vi "Sensor Calibration.vi"(5 "Error In":errorcluster) -> (15 "SubGP Slope":dbl, 16 "SubGP Intercept":dbl, 17 "Flow Slope":dbl, 18 "Flow Intercept":dbl, 19 "Error Out":errorcluster)   [LabVIEW 2020, in "MainVIs.lvlib"]
uses:
  MainVIs.lvlib
  <vilib>/Analysis/baseanly.llb/Mean (DBL).vi
  <vilib>/Analysis/NI_AALBase.lvlib
  SubVIs.lvlib
panel:
  out "SupraGP Slope":dbl
  out "SupraGP Intercept":dbl
  out "SupraGP Voltage":dbl
  out "Flow Voltage":dbl
  in  "Add Button HS":bool
  in  "Stop Button HS":bool
  out "SubGP Voltage":dbl
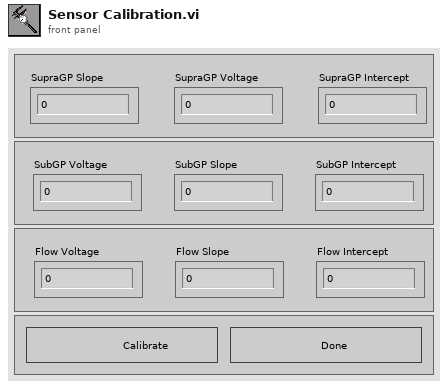
[diagram p1: front panel]
types:
  T1 = enum8{"Enabled", "Disabled", "Disabled and Grayed Out"}
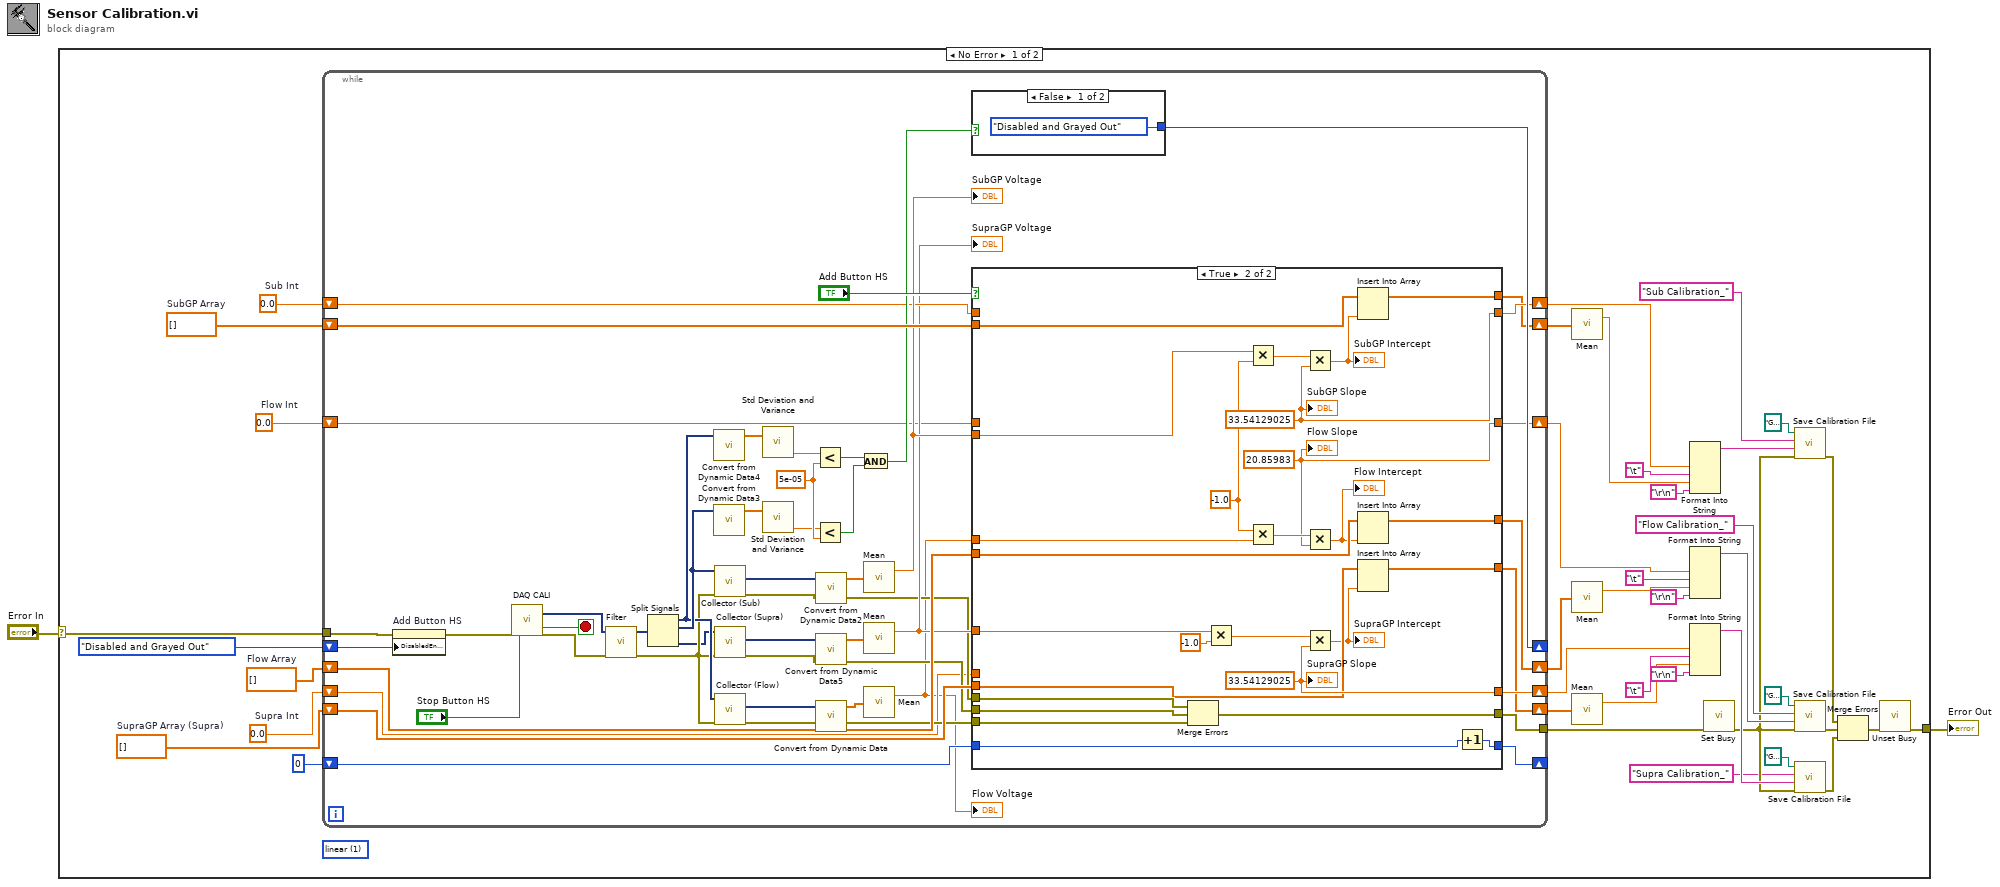
[diagram p0: block diagram]
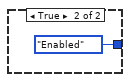
[diagram p2: hidden frame]
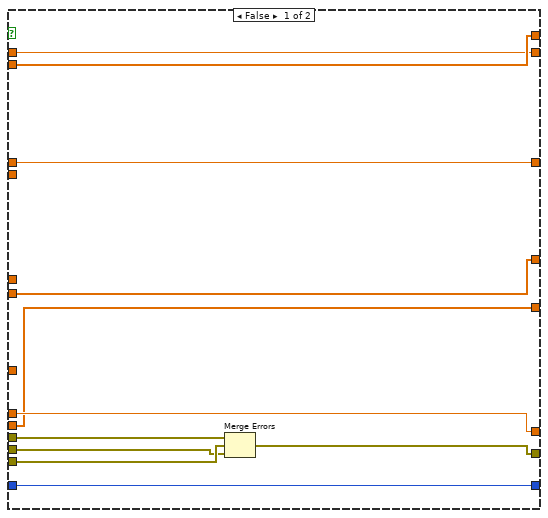
[diagram p3: hidden frame]
diagram:
  n1 = case shown="No Error" "Error In" {
    selector: "Error In" -> [w13 w131]
    tunnel: [w35 w131] -> w2
    frame No Error {
      w4 = 0.0  # Supra Int
      w11 = 0.0  # Flow Int
      w14 = 0.0  # Sub Int
      w17 = dbl[] []  # SupraGP Array (Supra)
      w40 = dbl[] []  # SubGP Array
      (unwired) 1 items=["nearest", "linear", "spline", "cubic Hermite", "Lagrange"] ("method")
      w42 = dbl[] []  # Flow Array
      n2 = while {
        tunnel: w13 -> [w78]
        shift-right: [w59] -> w12
        shift-left: w42 -> [w82]
        shift-right: [w83] -> _
        shift-left: 0 -> [w84]
        shift-right: [w60] -> w16
        shift-left: w40 -> [w79]
        shift-right: [w70] -> _
        shift-left: T1."Disabled and Grayed Out" ("Disabled") -> [w76]
        shift-right: [w62] -> w36
        shift-left: w14 -> [w61]
        shift-right: [w43] -> w3
        shift-left: w17 -> [w54]
        shift-right: [w50] -> w6
        shift-left: w4 -> [w49]
        shift-right: [w46] -> w8
        shift-left: w11 -> [w45]
        tunnel: [w44] -> w9
        stop <- w87 stop-if-true
        w69 = 5e-05
        n3 = property on="Add Button HS" class="Bool"(error in=w78, "DisabledEnum"=w76) -> (error out=w77:errorcluster)  [unwired: 1 in, 1 out]
        n4 = call "DAQ CALI"("error in"=w77, "stop (F)"="Stop Button HS") -> ("data"=w90:dynamicdata, "stopped"=w87:bool, "error out"=w91:errorcluster)  [unwired: 14 in, 1 out]
        n5 = call "Filter"("error in (no error)"=w91, "Signal"=w90) -> ("error out"=w58:errorcluster, "Filtered Signal"=w81:dynamicdata)  [unwired: 8 in]
        n6 = Split Signals(w81) -> (w63:dynamicdata, w68:dynamicdata, w48:dynamicdata)  [unwired: 4 in, 1 out]
        n7 = call "Convert from Dynamic Data4"("Dynamic Data Type"=w63) -> ("Array"=w67:dbl[])  [unwired: 3 in]
        n8 = call "Convert from Dynamic Data3"("Dynamic Data Type"=w68) -> ("Array"=w66:dbl[])  [unwired: 3 in]
        n9 = call "Collector (Sub)"("error in (no error)"=w58, "Signals"=w68) -> ("error out"=w51:errorcluster, "Collected Signals"=w80:dynamicdata)  [unwired: 8 in]
        n10 = call "Collector (Supra)"("error in (no error)"=w58, "Signals"=w48) -> ("error out"=w53:errorcluster, "Collected Signals"=w57:dynamicdata)  [unwired: 8 in]
        n11 = call "Collector (Flow)"("error in (no error)"=w58, "Signals"=w63) -> ("error out"=w52:errorcluster, "Collected Signals"=w86:dynamicdata)  [unwired: 8 in]
        n12 = call <vilib>:"Std Deviation and Variance.vi"("X"=w67) -> ("variance"=w64:dbl)  [unwired: 1 in, 2 out]
        n13 = call <vilib>:"Std Deviation and Variance.vi"("X"=w66) -> ("variance"=w65:dbl)  [unwired: 1 in, 2 out]
        n14 = Less?(x=w64, y=w69) -> (x < y?=w73:bool)
        n15 = Less?(x=w65, y=w69) -> (x < y?=w72:bool)
        n16 = call "Convert from Dynamic Data2"("Dynamic Data Type"=w80) -> ("Array"=w75:dbl[])  [unwired: 3 in]
        n17 = call "Convert from Dynamic Data5"("Dynamic Data Type"=w57) -> ("Array"=w56:dbl[])  [unwired: 3 in]
        n18 = call "Convert from Dynamic Data"("Dynamic Data Type"=w86) -> ("Array"=w85:dbl[])  [unwired: 3 in]
        n19 = And(x=w73, y=w72) -> (x .and. y?=w71:bool)
        n20 = call-poly <vilib>:"Mean.vi"("X"=w75) -> ("mean"=w74:dbl)  [unwired: 1 out]
        "SubGP Voltage" <- w74
        n21 = call-poly <vilib>:"Mean.vi"("X"=w56) -> ("mean"=w55:dbl)  [unwired: 1 out]
        "SupraGP Voltage" <- w55
        n22 = call-poly <vilib>:"Mean.vi"("X"=w85) -> ("mean"=w47:dbl)  [unwired: 1 out]
        "Flow Voltage" <- w47
        n23 = case shown="False" w71 {
          tunnel: [T1."Disabled and Grayed Out" ("Disabled") T1."Enabled" ("Disabled")] -> w70
          frame False {
          }
          frame True {
          }
        }
        n24 = case shown="True" "Add Button HS" {
          tunnel: [w97 w128] -> w44
          tunnel: w84 -> [w104 w130]
          tunnel: [w104 w129] -> w83
          tunnel: w82 -> [w103 w120]
          tunnel: [w103 w119] -> w59
          tunnel: w79 -> [w102 w121]
          tunnel: w74 -> [_ w127]
          tunnel: [w102 w122] -> w60
          tunnel: [w101 w125] -> w62
          tunnel: w61 -> [w101 _]
          tunnel: w55 -> [_ w111]
          tunnel: w54 -> [w94 w107]
          tunnel: w53 -> [w98 w113]
          tunnel: w52 -> [w99 w112]
          tunnel: w51 -> [w100 w124]
          tunnel: [w96 w108] -> w50
          tunnel: [w94 w106] -> w43
          tunnel: w49 -> [w96 _]
          tunnel: w47 -> [_ w117]
          tunnel: [w95 w114] -> w46
          tunnel: w45 -> [w95 _]
          frame False {
            n25 = Merge Errors(w100, w99, w98) -> (w97:errorcluster)
          }
          frame True {
            w108 = 33.54129025
            w114 = 20.85983 ("y")
            w118 = -1.0 ("y")
            w125 = 33.54129025
            n26 = Merge Errors(w124, w113, w112) -> (w128:errorcluster)
            n27 = Multiply(x=w111, y=-1.0) -> (x*y=w109:dbl)
            n28 = Multiply(x=w127, y=w118) -> (x*y=w126:dbl)
            n29 = Multiply(x=w118, y=w117) -> (x*y=w116:dbl)
            n30 = Multiply(x=w126, y=w125) -> (x*y=w123:dbl)
            "SubGP Intercept" <- w123
            n31 = Multiply(x=w116, y=w114) -> (x*y=w115:dbl)
            "Flow Intercept" <- w115
            n32 = Multiply(x=w109, y=w108) -> (x*y=w105:dbl)
            "SupraGP Intercept" <- w105
            n33 = Insert Into Array(array=w121, new element=w123) -> (w122:dbl[])  [unwired: 1 in]
            n34 = Insert Into Array(array=w120, new element=w115) -> (w119:dbl[])  [unwired: 1 in]
            n35 = Insert Into Array(array=w107, new element=w105) -> (w106:dbl[])  [unwired: 1 in]
            n36 = Increment(x=w130) -> (x+1=w129:i32)
            "Flow Slope" <- w114
            "SubGP Slope" <- w125
            "SupraGP Slope" <- w108
          }
        }
      }
      n37 = call-poly <vilib>:"Mean.vi"("X"=w16) -> ("mean"=w15:dbl)  [unwired: 1 out]
      n38 = call-poly <vilib>:"Mean.vi"("X"=w12) -> ("mean"=w7:dbl)  [unwired: 1 out]
      n39 = call-poly <vilib>:"Mean.vi"("X"=w3) -> ("mean"=w5:dbl)  [unwired: 1 out]
      n40 = Format Into String(w36, "\t", w15, "\r\n") -> (resulting string=w30:string)  [unwired: 3 in, 1 out]
      n41 = Format Into String(w8, "\t", w7, "\r\n") -> (resulting string=w25:string)  [unwired: 3 in, 1 out]
      n42 = Format Into String(w6, "\t", w5, "\r\n") -> (resulting string=w21:string)  [unwired: 3 in, 1 out]
      n43 = call <vilib>:"Set Busy.vi"("error in (no error)"=w9) -> ("error out"=w20:errorcluster)  [unwired: 9 in, 1 out]
      n44 = call "Save Calibration File.vi"("error in"=w20, "Calibration Values"=w30, "File Name"="Sub Calibration_", "Cali File Path"=path "G:/1-Booth Program Updated - 2019/Calibration Files/Sub Calibration.txt" ("file path (use dialog)")) -> ("error out"=w10:errorcluster)  [unwired: 7 in]
      n45 = call "Save Calibration File.vi"("error in"=w20, "Calibration Values"=w25, "File Name"="Flow Calibration_", "Cali File Path"=path "G:/1-Booth Program Updated - 2019/Calibration Files/Flow Calibration.txt" ("file path (use dialog)")) -> ("error out"=w28:errorcluster)  [unwired: 7 in]
      n46 = call "Save Calibration File.vi"("error in"=w20, "Calibration Values"=w21, "File Name"="Supra Calibration_", "Cali File Path"=path "G:/1-Booth Program Updated - 2019/Calibration Files/Supra Calibration.txt" ("file path (use dialog)")) -> ("error out"=w19:errorcluster)  [unwired: 7 in]
      n47 = Merge Errors(w10, w28, w19) -> (w32:errorcluster)
      n48 = call <vilib>:"Unset Busy.vi"("error in (no error)"=w32) -> ("error out"=w35:errorcluster)  [unwired: 10 in]
    }
    frame Error {
    }
  }
  "Error Out" <- w2
